vi "write.vi"(8 "error in (no error)":errorcluster, 10 "String to send":string, 11 "CEG4500 in":refnum<class "CEG4500.lvclass">) -> (0 "error out":errorcluster, 3 "CEG4500 out":refnum<class "CEG4500.lvclass">)   [LabVIEW 2013, in "CEG4500.lvclass"]
uses:
  CEG4500.lvclass
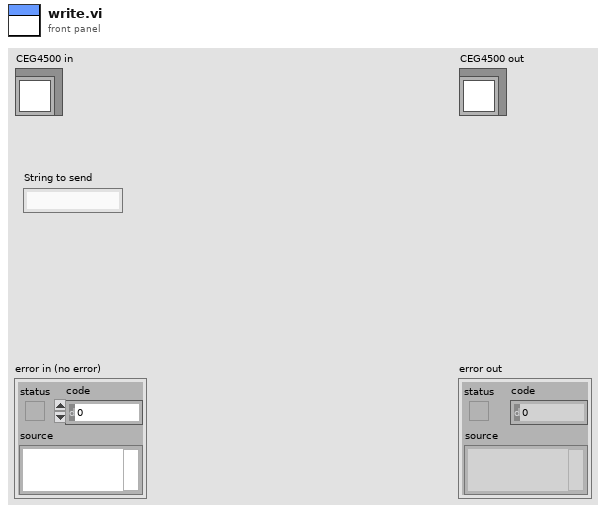
[diagram p1: front panel]
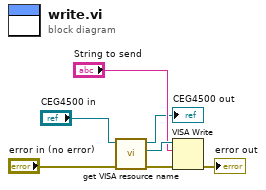
[diagram p0: block diagram]
diagram:
  n1 = call-dynamic "get VISA resource name.vi"("error in (no error)"="error in (no error)", "DeviceInterface (Eingang)"="CEG4500 in") -> ("error out"=w2:errorcluster, "VISA resource name"=w7:refnum<visa-resource-name>, "DeviceInterface (Ausgang)"=→"CEG4500 out":refnum<class "CEG4500.lvclass">)  [unwired: 7 in]
  n2 = VISA Write(VISA resource name=w7, write buffer="String to send", error in (no error)=w2) -> (error out=→"error out":errorcluster)  [unwired: 2 out]
